vi "get button states for selection list.vi"(9 "not present item indexes":i32[](array[numeric]), 10 "selected items":i32[](array[numeric]), 11 "reserved item indexes":i32[](array[numeric])) -> (2 "remove enable":bool, 3 "add enable":bool)   [LabVIEW 2016, in "FPGA Addon System Explorer.lvlib"]
uses:
  FPGA Addon System Explorer.lvlib
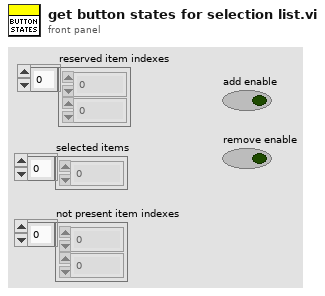
[diagram p1: front panel]
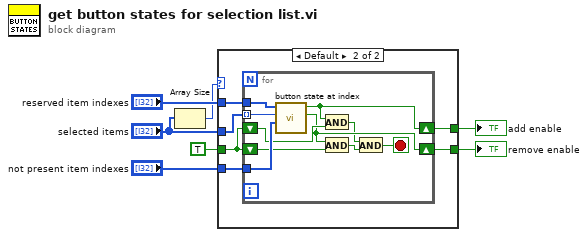
[diagram p0: block diagram]
diagram:
  n1 = Array Size(array="selected items") -> (size(s)=w1:i32)
  n2 = case shown="Default" w1 {
    tunnel: [_ w13] -> w7
    tunnel: [_ w12] -> w6
    tunnel: "reserved item indexes" -> [_ w11]
    tunnel: TRUE -> [_ w10]
    tunnel: "not present item indexes" -> [_ w9]
    tunnel: "selected items" -> [_ w8]
    frame 0 {
    }
    frame Default {
      n3 = for {
        tunnel: w8 -> [w21] mode=indexing
        tunnel: w9 -> [w23]
        shift-right: [w20] -> w13
        shift-left: w10 -> [w19]
        shift-right: [w18] -> w12
        shift-left: w10 -> [w17]
        tunnel: w11 -> [w22]
        stop <- w16 stop-if-true
        n4 = call "button state at index.vi"("not present item indexes"=w23, "index"=w21, "reserved item indexes"=w22) -> ("remove enable"=w18:bool, "add enable"=w20:bool)  [unwired: 7 in]
        n5 = And(x=w20, y=w19) -> (x .and. y?=w15:bool)
        n6 = And(x=w18, y=w17) -> (x .and. y?=w14:bool)
        n7 = And(x=w15, y=w14) -> (x .and. y?=w16:bool)
      }
    }
  }
  "add enable" <- w7
  "remove enable" <- w6
